vi "LSX Get Analog Inputs2.vi"(7 "plV24":i32, 8 "error in (no error)":errorcluster, 9 "plMV":i32, 10 "plPT100":i32, 11 "lLSID":i32) -> (0 "error out":errorcluster, 1 "plMV out":i32, 2 "plPT100 out":i32, 3 "function return":i32, 5 "plV24 out":i32)   [LabVIEW 2016, in "Tango_DLL.lvlib"]
doc: "TANGOAPI int TANGOCALL LSX_GetAnalogInputs2 (int lLSID, int *plPT100, int *plMV, int *plV24);"
uses:
  Tango_DLL.lvlib
  2017/Microscope Control/Device Library/Stages/Marzhauser/SCAN IM 120 x 80/Tango DLL VIs/Tango_DLL.dll
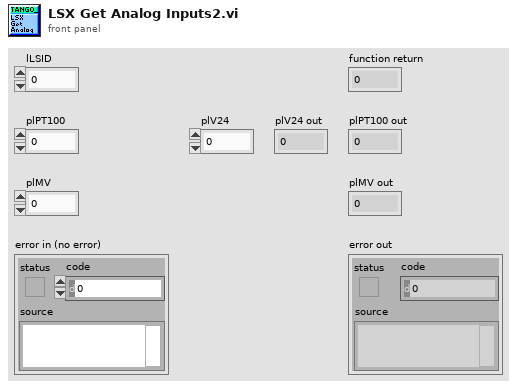
[diagram p1: front panel]
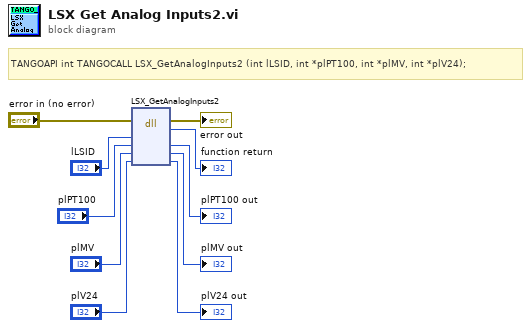
[diagram p0: block diagram]
diagram:
  # "TANGOAPI int TANGOCALL LSX_GetAnalogInputs2 (int lLSID, int *plPT100, int *plMV, int *plV24);"
  n1 = dll-call lib="C:/Users/4PiSMS/Documents/Microscope Control/2017/Microscope Control/Device Library/Stages/Marzhauser/SCAN IM 120 x 80/Tango DLL VIs/Tango_DLL.*" fn="LSX_GetAnalogInputs2"(error in="error in (no error)", "lLSID"="lLSID", "plPT100"="plPT100", "plMV"="plMV", "plV24"="plV24") -> (error out=→"error out":errorcluster, →"function return":i32, "plPT100"=→"plPT100 out":i32, "plMV"=→"plMV out":i32, "plV24"=→"plV24 out":i32)  [unwired: 3 in, 1 out]
